vi "超标留样启动留样.vi"(8 "error in (no error)":errorcluster) -> (0 "error out":errorcluster)   [LabVIEW 2016, in "超标留样集成.lvlib" / "德润DR803M超标留样.lvlib"]
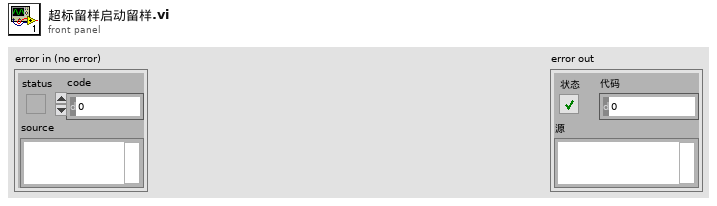
[diagram p1: front panel]
types:
  T1 = typedef "超标留样集成.lvlib/德润DR803M超标留样.lvlib/typedef.ctl" = cluster{"枚举":enum16{"open", "read", "write", "close", "write_register"}, "写入内容":string, "data_in":cluster{"write_coil_in":cluster{"address":u16, "value":bool}, "write_register_in":cluster{"address":u16, "values":u16[]}, "read_register_in":cluster{"starting address":u16, "quantity":u16}}}
  T2 = enum16{"open", "read", "write", "close", "write_register"}
  T3 = enum16{"停止", "运行", "系统初始化-2", "系统初始化-3", "初始化失败"}
  T4 = cluster{"仪器时间":timestamp, "工作状态":u16, "工作进程":u16, "采样模式":u16, "采样瓶数":dbl, "当前瓶号":dbl, "设定平行样数":dbl, "已采平行样":dbl, "设定每瓶采样次数":dbl, "已采次数":dbl, "当前瓶采样量":dbl, "瞬时流量":dbl, "累积流量":dbl, "混匀桶已采次数":dbl, "COD":dbl, "NH3N":dbl, "门状态":u16, "采样泵使能":dbl, "采样泵方向":dbl, "导流电机使能":dbl, "导流电机方向":dbl, "阀A":dbl, "阀B":dbl, "阀C":dbl, "外置泵":dbl, "预留":dbl}
  T5 = cluster{"采样器状态":enum16{"停止", "运行", "系统初始化-2", "系统初始化-3", "初始化失败"}, "仪器时间":timestamp, "留样结果":bool, "工作模式":u16, "当前瓶号":u16, "平行样数":u16, "采样瓶数":u16, "设定每瓶采样次数":u16, "每瓶采样量":u16, "当前进程":u16, "当前瓶已采次数":u16, "留样中":bool}
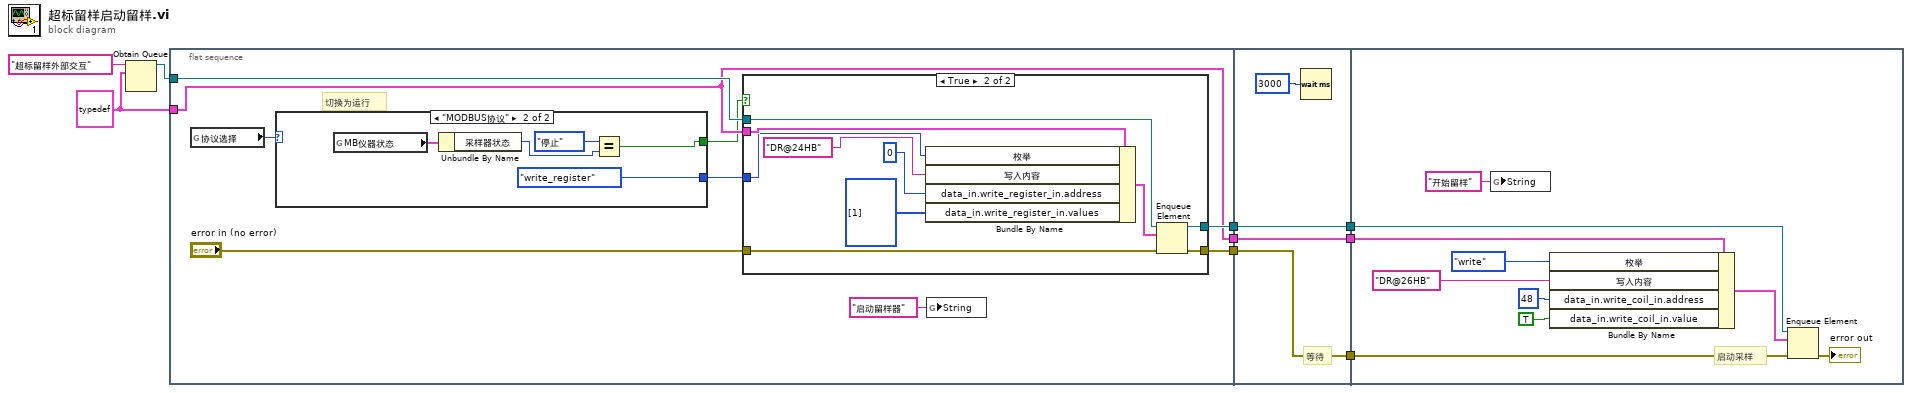
[diagram p0: block diagram]
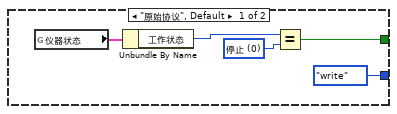
[diagram p3: hidden frame]
diagram:
  w3 = T1 {"枚举"=enum."open", "写入内容"="超标留样", "data_in"={"write_coil_in"={"address"=0, "value"=FALSE}, "write_register_in"={"address"=0, "values"=[]}, "read_register_in"={"starting address"=0, "quantity"=0}}}
  n1 = Obtain Queue(name (unnamed)="超标留样外部交互" ("名称（未命名）"), element data type=w3) -> (queue out=w6:refnum<queue>)  [unwired: 3 in, 2 out]
  n2 = flat-sequence {
    tunnel: [w16] -> w8
    tunnel: w6 -> [w18]
    tunnel: [w15] -> w4
    tunnel: w3 -> [w14]
    tunnel: [w14] -> w1
    tunnel: [w43] -> w9
    tunnel: w8 -> [w43]
    tunnel: [w42] -> w5
    tunnel: w4 -> [w42]
    tunnel: [w41] -> w2
    tunnel: w1 -> [w41]
    tunnel: w9 -> [w51]
    tunnel: w5 -> [w52]
    tunnel: w2 -> [w48]
    frame #0 {
      # "切换为运行"
      n3 = global read "超标留样全局.vi" "协议选择"() -> (w13:enum16{"原始协议", "MODBUS协议"})
      n4 = case shown="\"MODBUS协议\"" w13 {
        tunnel: [T2."write" ("枚举") T2."write_register" ("枚举")] -> w12
        tunnel: [w31 w36] -> w11
        frame "原始协议", Default {
          w32 = u16 0 items=["停止", "运行", "系统初始化"] ("工作状态")
          n5 = global read "超标留样全局.vi" "仪器状态"() -> (w34:T4)
          n6 = Unbundle By Name(w34) -> ("工作状态"=w33:u16)
          n7 = Equal?(x=w33, y=w32) -> (x = y?=w31:bool)
        }
        frame "MODBUS协议" {
          n8 = global read "超标留样全局.vi" "MB仪器状态"() -> (w39:T5)
          n9 = Unbundle By Name(w39) -> ("采样器状态"=w38:T3)
          n10 = Equal?(x=T3."停止" ("采样器状态"), y=w38) -> (x = y?=w36:bool)
        }
      }
      n11 = case shown="True" w11 {
        tunnel: w18 -> [w20 w30]
        tunnel: "error in (no error)" -> [w19 w29]
        tunnel: [w19 w27] -> w16
        tunnel: [w20 w26] -> w15
        tunnel: w14 -> [_ w25]
        tunnel: w12 -> [_ w24]
        frame False {
        }
        frame True {
          n12 = Bundle By Name(cluster=w25, "枚举"=w24, "写入内容"="DR@24HB", "data_in.write_register_in.address"=u16 0, "data_in.write_register_in.values"=u16[] [1]) -> (w21:T1)
          n13 = Enqueue Element(queue=w30, element=w21, error in (no error)=w29) -> (queue out=w26:refnum<queue>, error out=w27:errorcluster)  [unwired: 1 in, 1 out]
        }
      }
      n14 = global write "超标留样全局.vi" "String"("启动留样器" ("String")) -> ()
    }
    frame #1 {
      # "等待"
      n15 = Wait (ms)(milliseconds to wait=u32 3000 ("等待时间（毫秒）")) -> ()  [unwired: 1 out]
    }
    frame #2 {
      # "启动采样"
      n16 = global write "超标留样全局.vi" "String"("开始留样" ("String")) -> ()
      n17 = Bundle By Name(cluster=w48, "枚举"=enum16{"open", "read", "write", "close"}."write" ("STEP"), "写入内容"="DR@26HB", "data_in.write_coil_in.address"=u16 48, "data_in.write_coil_in.value"=TRUE) -> (w54:T1)
      n18 = Enqueue Element(queue=w52, element=w54, error in (no error)=w51) -> (error out=→"error out":errorcluster)  [unwired: 1 in, 2 out]
    }
  }
